vi "WLAN - niVST - RFSG - Init.vi"(11 "RFSG Handle":string) -> (0 "error out":errorcluster, 3 "RFSG handle out":refnum<k15>)   [LabVIEW 2012]
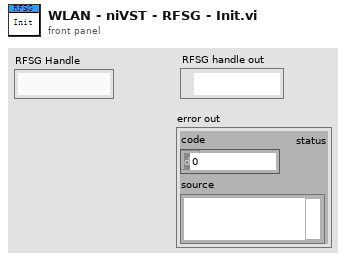
[diagram p1: front panel]
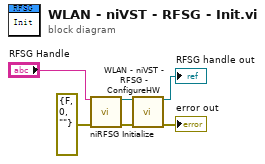
[diagram p0: block diagram]
diagram:
  n1 = call <instrlib>:"niRFSG Initialize.vi"("resource name"="RFSG Handle", "error in"=errorcluster {"status"=FALSE, "code"=0, "source"=""}) -> ("instrument handle"=w5:refnum<k15>, "error out"=w6:errorcluster)  [unwired: 12 in]
  n2 = call "WLAN - niVST - RFSG - ConfigureHW.vi"("instrument handle"=w5, "error in"=w6) -> ("instrument handle"=→"RFSG handle out":refnum<k15>, "error out"=→"error out":errorcluster)  [unwired: 12 in]
